vi "Connect.vi"(8 "error in (no error)":errorcluster, 11 "Ultimus V in":refnum<class "Ultimus V.lvclass">) -> (0 "error out":errorcluster, 3 "Ultimus V out":refnum<class "Ultimus V.lvclass">)   [LabVIEW 2019, in "Ultimus V.lvclass"]
uses:
  Ultimus V.lvclass
  Ultimus V.lvclass/Ultimus V.ctl
  Drivers/EFD Ultimus V/EFD Ultimus V.lvlib
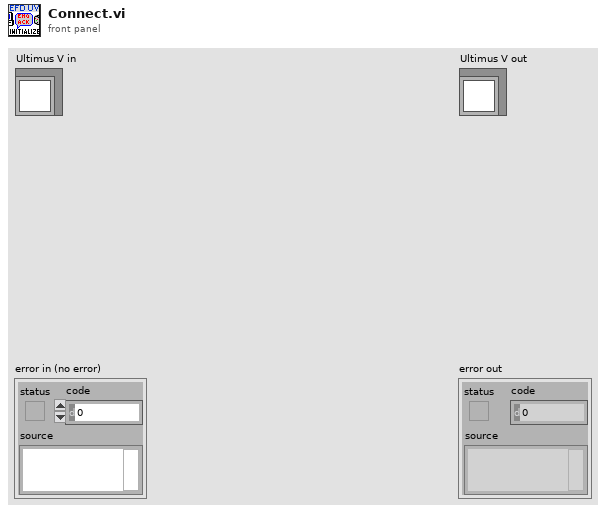
[diagram p1: front panel]
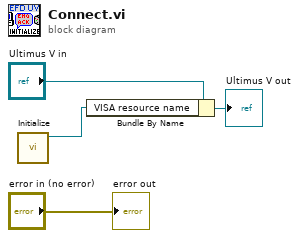
[diagram p0: block diagram]
diagram:
  n1 = call "Initialize.vi"() -> ("VISA resource name out"=w1:refnum<visa-resource-name>)  [unwired: 10 in, 1 out]
  n2 = Bundle By Name(cluster="Ultimus V in", "VISA resource name"=w1) -> (→"Ultimus V out":refnum<class "Ultimus V.lvclass">)
  "error out" <- "error in (no error)"
